vi "Configure List Step Parameters.vi"(0 "VISA resource name":refnum<visa-resource-name>, 1 "Step Number (1)":dbl=1.0 min=1.0 max=84.0 step=1.0 format="%.0g", 5 "Step Level (1)":dbl=1.0 min=1.0 max=240.0 step=0.01 format="%.4g", 7 "Step Width (1)":dbl=1.0 min=2e-05 max=3600.0 step=1.0 format="%.6g", 9 "Step Slew Rate (1)":dbl=1.0 min=0.0001 max=65536.0 step=0.0001 format="%.4g", 11 "error in (no error)":errorcluster) -> (4 "VISA resource name out":refnum<visa-resource-name>, 15 "error out":errorcluster)   [LabVIEW 2018, in "BK Precision 8600 Series.lvlib"]
doc: "Configures the step parameters of a list file for list mode operation. Use <b>Configure List Operation.vi</b> first to setup list parameters before configuring step parameters.\n\nNote: List mode is only available for CC mode."
uses:
  <instrlib>/BK Precision 8600 Series/BK Precision 8600 Series.lvlib
panel:
  # "s"
  # "A"
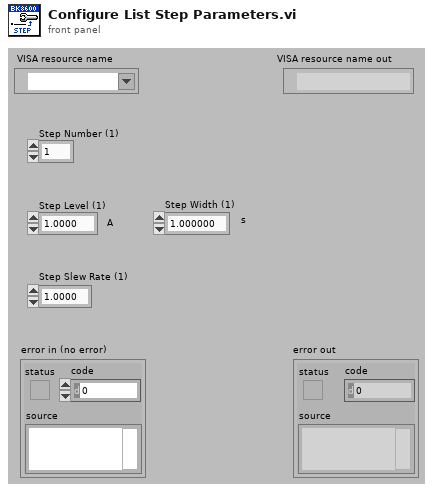
[diagram p1: front panel]
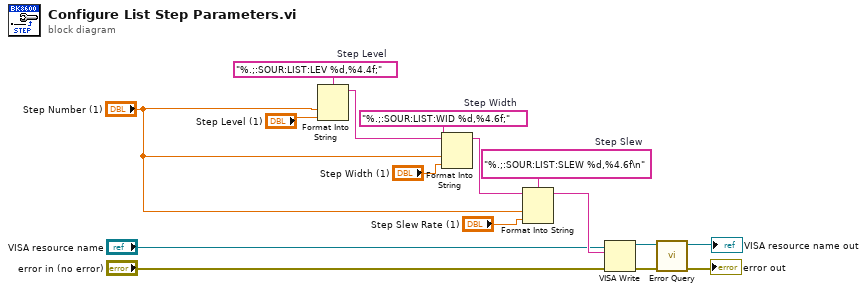
[diagram p0: block diagram]
diagram:
  w9 = "%.;:SOUR:LIST:LEV %d,%4.4f;"  # Step Level
  w11 = "%.;:SOUR:LIST:SLEW %d,%4.6f\n"  # Step Slew
  w12 = "%.;:SOUR:LIST:WID %d,%4.6f;"  # Step Width
  n1 = Format Into String(format string=w9, "Step Number (1)", "Step Level (1)") -> (resulting string=w8:string)  [unwired: 2 in, 1 out]
  n2 = Format Into String(format string=w12, initial string=w8, "Step Number (1)", "Step Width (1)") -> (resulting string=w10:string)  [unwired: 1 in, 1 out]
  n3 = Format Into String(format string=w11, initial string=w10, "Step Number (1)", "Step Slew Rate (1)") -> (resulting string=w7:string)  [unwired: 1 in, 1 out]
  n4 = VISA Write(VISA resource name="VISA resource name", write buffer=w7, error in (no error)="error in (no error)") -> (VISA resource name out=w15:refnum<visa-resource-name>, error out=w16:errorcluster)  [unwired: 1 out]
  n5 = call <instrlib>:"Error Query.vi"("error in (no error)"=w16, "VISA resource name"=w15) -> ("error out"=→"error out":errorcluster, "VISA resource name out"=→"VISA resource name out":refnum<visa-resource-name>)  [unwired: 6 in, 2 out]
